vi "Ctx Get.vi"(7 "path override":path, 8 "error in (no error)":errorcluster, 10 "option_":i32, 11 "context_":u32) -> (0 "error out":errorcluster, 3 "context_ out":u32)   [LabVIEW 2025, in "LibZMQ.lvlib"]
doc: "ZMQ_EXPORT int zmq_ctx_get (void *context_, int option_);"
uses:
  LibZMQ.lvlib
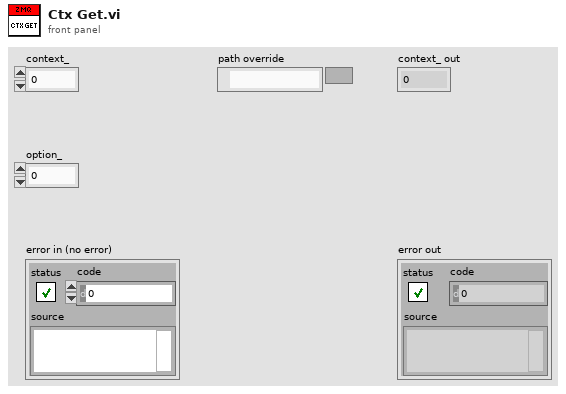
[diagram p1: front panel]
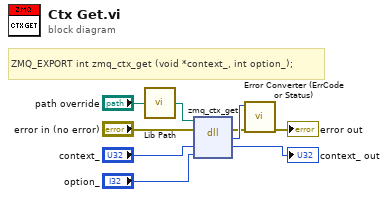
[diagram p0: block diagram]
diagram:
  # "ZMQ_EXPORT int zmq_ctx_get (void *context_, int option_);"
  n1 = call "Lib Path.vi"("path override"="path override") -> ("lib path"=w1:path)
  n2 = dll-call lib="C:/LV/LibZMQ/libzmq/lv_x86/bin/Release/libzmq-v143-mt-4_3_6.*" fn="zmq_ctx_get"(path in=w1, error in="error in (no error)", "context_"="context_", "option_"="option_") -> (error out=w4:errorcluster, "return type"=w9:i32, "context_"=→"context_ out":u32)  [unwired: 2 in, 1 out]
  n3 = call "Error Converter (ErrCode or Status).vi"("error in (no error)"=w4, "error code"=w9) -> ("error out"=→"error out":errorcluster)  [unwired: 9 in]
